vi "TEMP ON.vi"(6 "ScanQ in":refnum<queue>, 7 "element in":T2 {"Output's Control Loop (1:1)" items=["1"=1, "2"=2]; "Data Source (0:Kelvin)" items=["Kelvin", "Celsius", "Sensor Units"]; "Input (0:A)" items=["A", "B", "C", "D", "D2", "D3", "D4", "D5"]; "Configure Control Parameters (0: Configure)" items=["Configure", "Don't Configure"]; "Serial Configuration"."Flow Control" items=["None", "XON/XOFF", "RTS/CTS", "XON/XOFF & RTS/CTS", "DTR/DSR", "XON/XOFF & DTR/DSR"]; "Serial Configuration"."Stop Bits" items=["1.0"=10, "1.5"=15, "2.0"=20]; "Serial Configuration"."Data Bits" items=["7"=7, "8"=8]; "Serial Configuration"."Parity" items=["None", "Odd", "Even", "Mark", "Space"]; "Serial Configuration"."Baud Rate" items=["300"=300, "600"=600, "1200"=1200, "2400"=2400, "4800"=4800, "9600"=9600, "19200"=19200, "38400"=38400, "57600"=57600]; "Target Temp (K)" format="%.5f"; "Input (0:None)" items=["None", "A", "B", "C", "D", "D2", "D3", "D4", "D5"]; "Mode (0:Off)" items=["Off", "Closed Loop PID", "Zone", "Open Loop"]; "Heater Out Display (1:Current)" items=["Current"=1, "Power"=2]; "Max Current (0:User Specified)" items=["User Specified", "0.707 A", "1.0 A", "1.141 A", "2.0 A"]; "Heater Resistance (1:25 Ohms)" items=["25 Ohms"=1, "50 Ohms"=2]; "Max User Current (2.000)" format="%.3f"; "Gain (P) (50.0)" format="%.1f"; "Reset (I) (20.0)" format="%.1f"; "Rate (D) (0.0 %)" format="%.1f"; "Manual Output (0.00 %)" format="%.2f"; "Range (0:Off)" items=["Off", "Range 1 (On)", "Range 2", "Range 3", "Range 4", "Range 5"]}, 8 "error in (no error)":errorcluster, 9 "Field and Temp Range":T1={"VISA (Magnet)"="COM4", "Fields(T)"=[], "Temps(K)"=[], "VISA (Temp) "="COM1"}, 10 "TempQ in":refnum<queue>, 11 "VISA Refnum in":refnum<visa-resource-name>) -> (0 "error out":errorcluster, 1 "element out":T2 {"Output's Control Loop (1:1)" items=["1"=1, "2"=2]; "Data Source (0:Kelvin)" items=["Kelvin", "Celsius", "Sensor Units"]; "Input (0:A)" items=["A", "B", "C", "D", "D2", "D3", "D4", "D5"]; "Configure Control Parameters (0: Configure)" items=["Configure", "Don't Configure"]; "Serial Configuration"."Flow Control" items=["None", "XON/XOFF", "RTS/CTS", "XON/XOFF & RTS/CTS", "DTR/DSR", "XON/XOFF & DTR/DSR"]; "Serial Configuration"."Stop Bits" items=["1.0"=10, "1.5"=15, "2.0"=20]; "Serial Configuration"."Data Bits" items=["7"=7, "8"=8]; "Serial Configuration"."Parity" items=["None", "Odd", "Even", "Mark", "Space"]; "Serial Configuration"."Baud Rate" items=["300"=300, "600"=600, "1200"=1200, "2400"=2400, "4800"=4800, "9600"=9600, "19200"=19200, "38400"=38400, "57600"=57600]; "Target Temp (K)" format="%.5f"; "Input (0:None)" items=["None", "A", "B", "C", "D", "D2", "D3", "D4", "D5"]; "Mode (0:Off)" items=["Off", "Closed Loop PID", "Zone", "Open Loop"]; "Heater Out Display (1:Current)" items=["Current"=1, "Power"=2]; "Max Current (0:User Specified)" items=["User Specified", "0.707 A", "1.0 A", "1.141 A", "2.0 A"]; "Heater Resistance (1:25 Ohms)" items=["25 Ohms"=1, "50 Ohms"=2]; "Max User Current (2.000)" format="%.3f"; "Gain (P) (50.0)" format="%.1f"; "Reset (I) (20.0)" format="%.1f"; "Rate (D) (0.0 %)" format="%.1f"; "Manual Output (0.00 %)" format="%.2f"; "Range (0:Off)" items=["Off", "Range 1 (On)", "Range 2", "Range 3", "Range 4", "Range 5"]}, 2 "TempQ out":refnum<queue>, 3 "VISA Refnum out":refnum<visa-resource-name>, 4 "ScanQ out":refnum<queue>, 5 "Setpoint":dbl format="%.5f")   [LabVIEW 2025]
uses:
  Downloads/OneDrive_2025-09-03/Instrument Controls/Temp Cntrl.ctl
  <instrlib>/Lake Shore 350/Lake Shore 350.lvlib
  STM-Auto-Project/QMH CTLS/Scan_Params (QMH).ctl
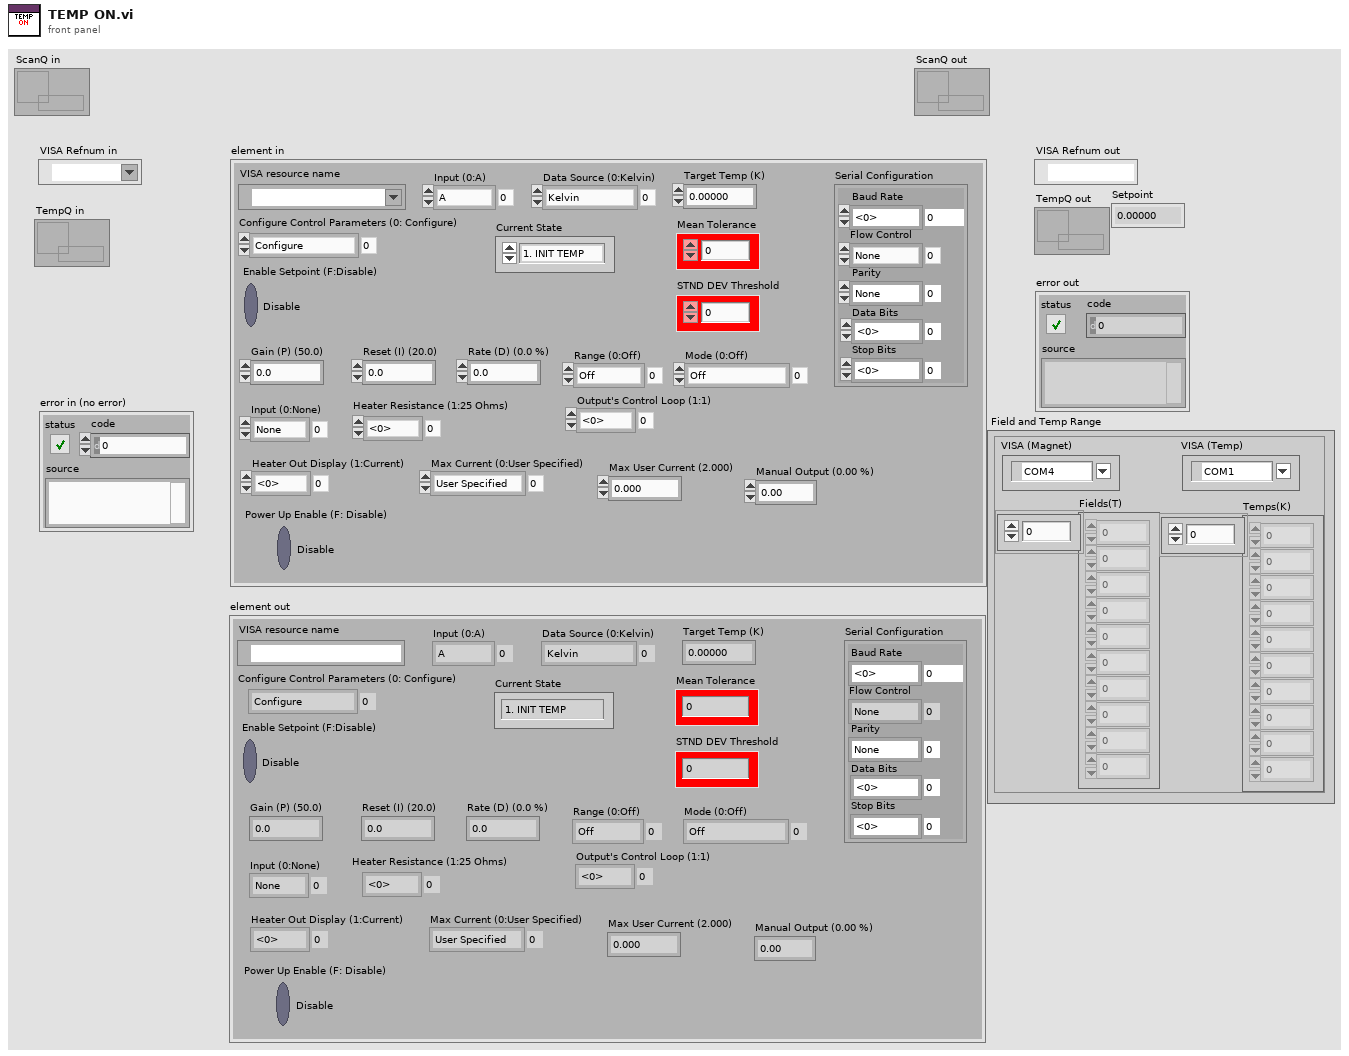
[diagram p1: front panel]
types:
  T1 = cluster{"VISA (Magnet)":refnum<visa-resource-name>, "Fields(T)":dbl[], "Temps(K)":dbl[], "VISA (Temp) ":refnum<visa-resource-name>}
  T2 = typedef "Temp Cntrl.ctl" = cluster{"Range (0:Off)":u16, "Manual Output (0.00 %)":dbl, "Rate (D) (0.0 %)":dbl, "Reset (I) (20.0)":dbl, "Gain (P) (50.0)":dbl, "Power Up Enable (F: Disable)":bool, "Max User Current (2.000)":dbl, "Heater Resistance (1:25 Ohms)":u16, "Max Current (0:User Specified)":u16, "Heater Out Display (1:Current)":u16, "Mode (0:Off)":u16, "Input (0:None)":u16, "Target Temp (K)":dbl, "Serial Configuration":cluster{"Baud Rate":u32, "Parity":u16, "Data Bits":u16, "Stop Bits":u16, "Flow Control":u16}, "VISA resource name":refnum<visa-resource-name>, "Configure Control Parameters (0: Configure)":u16, "Enable Setpoint (F:Disable)":bool, "Input (0:A)":u16, "Data Source (0:Kelvin)":u16, "Output's Control Loop (1:1)":u16, "STND DEV Threshold ":dbl, "Mean Tolerance ":dbl, "Current State":enum16{"1. INIT TEMP", "2. TC ON", "3. POLL_TEMPS", "4. TEMP_STAB", "5. TC IDLE", "6. APPLY NEXT TEMP", "7. TC OFF (Reset)"}}
  T3 = enum16{"1. BIAS", "2. INIT_SCAN", "3. SCAN_IDLE", "4. INTER_SCAN", "5. NEW_COORDS_&_FRAME", "6. FINAL_SCAN", "7. POLL BIAS ", "8. Z-CONT.", "9. STOP"}
  T4 = typedef "Scan_Params (QMH).ctl" = cluster{"Setpoint (I)":dbl[], "Bias (V)":dbl[], "Number of scans":u8, "Port number (3364)":u32, "Avoid zero threshold (V)":dbl, "Current State":enum16{"1. BIAS", "2. INIT_SCAN", "3. SCAN_IDLE", "4. INTER_SCAN", "5. NEW_COORDS_&_FRAME", "6. FINAL_SCAN", "7. POLL BIAS ", "8. Z-CONT.", "9. STOP"}}
  T5 = enum16{"1. INIT TEMP", "2. TC ON", "3. POLL_TEMPS", "4. TEMP_STAB", "5. TC IDLE", "6. APPLY NEXT TEMP", "7. TC OFF (Reset)"}
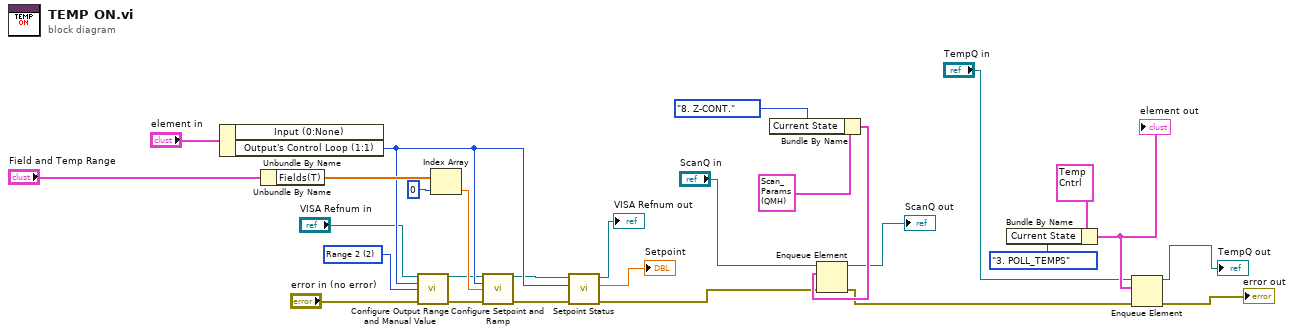
[diagram p0: block diagram]
diagram:
  w11 = u16 2 items=["Off", "Range 1 (On)", "Range 2", "Range 3", "Range 4", "Range 5"] ("Range (0:Off)")
  n1 = Unbundle By Name("element in") -> ("Output's Control Loop (1:1)"=w24:u16)  [unwired: 1 out]
  n2 = Unbundle By Name("Field and Temp Range") -> ("Fields(T)"=w25:dbl[])
  n3 = call <instrlib>:"Configure Output Range and Manual Value.vi"("VISA resource name"="VISA Refnum in", "Output (1:1)"=w24, "Range (0:Off)"=w11, "error in (no error)"="error in (no error)") -> ("VISA resource name out"=w20:refnum<visa-resource-name>, "error out"=w21:errorcluster)  [unwired: 10 in]
  n4 = Index Array(array=w25, index=0) -> (element=w26:dbl)
  n5 = call <instrlib>:"Configure Setpoint and Ramp.vi"("VISA resource name"=w20, "Output's Control Loop (1:1)"=w24, "Setpoint (0.00000)"=w26, "error in (no error)"=w21) -> ("VISA resource name out"=w23:refnum<visa-resource-name>, "error out"=w22:errorcluster)  [unwired: 10 in]
  n6 = call <instrlib>:"Setpoint Status.vi"("error in (no error)"=w22, "Output (1:1)"=w24, "VISA resource name"=w23) -> ("error out"=w3:errorcluster, "Setpoint"=→"Setpoint":dbl, "VISA resource name out"=→"VISA Refnum out":refnum<visa-resource-name>)  [unwired: 6 in]
  n7 = Bundle By Name(cluster=T4 {"Setpoint (I)"=[], "Bias (V)"=[], "Number of scans"=1, "Port number (3364)"=3364, "Avoid zero threshold (V)"=0.004999999888241291, "Current State"=enum."1. BIAS"} ("element"), "Current State"=T3."8. Z-CONT.") -> (w4:T4)
  n8 = Enqueue Element(queue="ScanQ in", element=w4, error in (no error)=w3) -> (queue out=→"ScanQ out":refnum<queue>, error out=w2:errorcluster)  [unwired: 1 in, 1 out]
  n9 = Bundle By Name(cluster=T2 {"Range (0:Off)"=0, "Manual Output (0.00 %)"=0.0, "Rate (D) (0.0 %)"=0.0, "Reset (I) (20.0)"=20.0, "Gain (P) (50.0)"=50.0, "Power Up Enable (F: Disable)"=FALSE, "Max User Current (2.000)"=2.0, "Heater Resistance (1:25 Ohms)"=1, "Max Current (0:User Specified)"=0, "Heater Out Display (1:Current)"=1, "Mode (0:Off)"=1, "Input (0:None)"=4, "Target Temp (K)"=5.0, "Serial Configuration"={"Baud Rate"=57600, "Parity"=1, "Data Bits"=7, "Stop Bits"=10, "Flow Control"=0}, "VISA resource name"="", "Configure Control Parameters (0: Configure)"=0, "Enable Setpoint (F:Disable)"=FALSE, "Input (0:A)"=3, "Data Source (0:Kelvin)"=0, "Output's Control Loop (1:1)"=2, "STND DEV Threshold "=0.1, "Mean Tolerance "=0.02, "Current State"=enum."1. INIT TEMP"} ("element"), "Current State"=T5."3. POLL_TEMPS") -> (w17:T2)
  "element out" <- w17
  n10 = Enqueue Element(queue="TempQ in", element=w17, error in (no error)=w2) -> (queue out=→"TempQ out":refnum<queue>, error out=→"error out":errorcluster)  [unwired: 1 in, 1 out]
